vi "BMark_Create Tree.vi"(8 "error in (no error)":errorcluster, 9 "GroupByVI":bool, 10 "TreeRef":refnum<vi>, 11 "Bookmark info":T1[](array[typedef])) -> (0 "error out":errorcluster)   [LabVIEW 2017]
uses:
  controls/BMark_Bookmark Data.ctl
  controls/BMark_VI_Identifier.ctl
  <vilib>/addons/analyzer/_analyzerctrls.llb/VIAnCtl Analysis App Info.ctl
  globals/BMark_User Visible Strings.vi
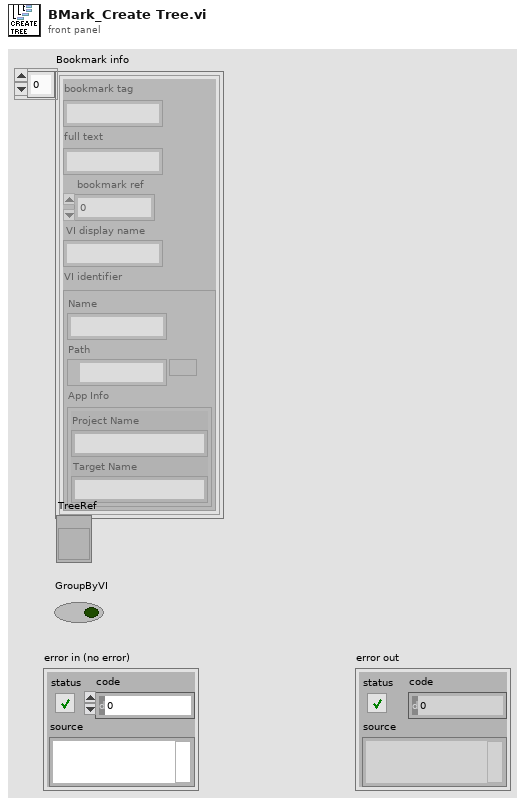
[diagram p1: front panel]
types:
  T1 = typedef "BMark_Bookmark Data.ctl" = cluster{"bookmark tag":string, "full text":string, "bookmark ref":i32, "VI display name":string, "VI identifier":T2}
  T2 = typedef "BMark_VI_Identifier.ctl" = cluster{"Name":string, "Path":path, "App Info":T3}
  T3 = typedef "VIAnCtl Analysis App Info.ctl" = cluster{"Project Name":string, "Target Name":string}
  T4 = enum8{"Enabled", "Disabled", "Disabled and Grayed Out"}
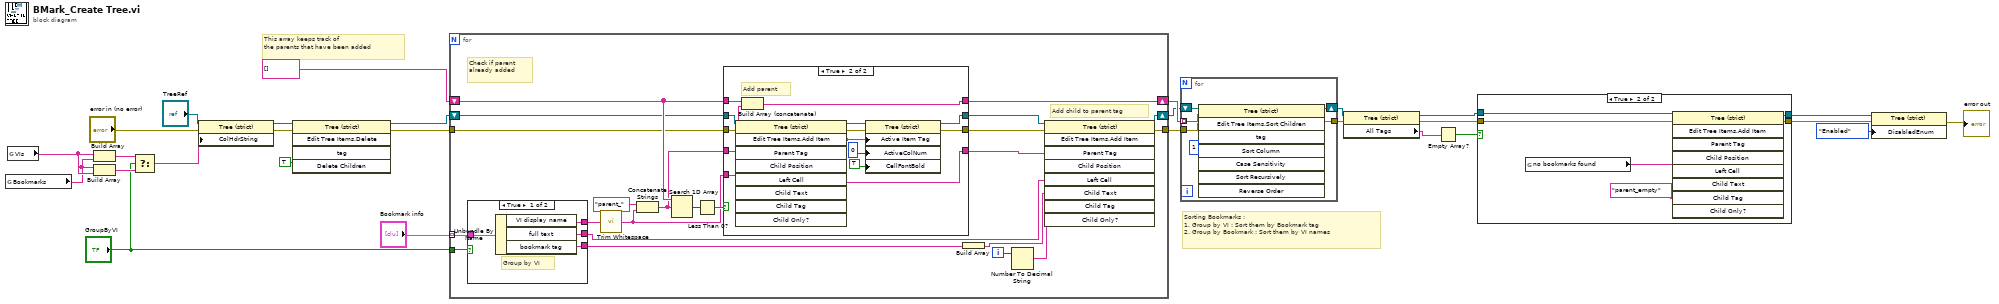
[diagram p0: block diagram]
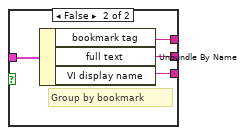
[diagram p2: hidden frame]
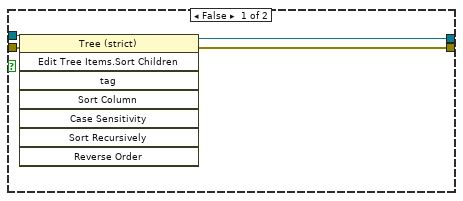
[diagram p4: hidden frame]
diagram:
  # "Sorting Bookmarks :\n1. Group by VI : Sort them by Bookmark tag\n2. Group by Bookmark : Sort them by VI names"
  # "This array keeps track of \nthe parents that have been added"
  n1 = global read "BMark_User Visible Strings.vi" "Bookmarks"() -> (w5:string)
  n2 = global read "BMark_User Visible Strings.vi" "VIs"() -> (w6:string)
  n3 = Build Array(w6, w5) -> (w18:string[])
  n4 = Build Array(w5, w6) -> (w17:string[])
  n5 = Select(t=w18, s="GroupByVI", f=w17) -> (s? t:f=w16:string[])
  n6 = property class="Tree (strict)"(reference="TreeRef", error in="error in (no error)", "ColHdrString"=w16) -> (reference out=w11:refnum<vi>, error out=w12:errorcluster)
  n7 = invoke class="Tree (strict)" method="Edit Tree Items.Delete"(reference=w11, error in=w12, "Delete Children"=TRUE ("Delete Children?")) -> (reference out=w26:refnum<vi>, error out=w27:errorcluster)  [unwired: 2 in, 3 out]
  n8 = for {
    tunnel: "Bookmark info" -> [w50] mode=indexing
    shift-right: [w46] -> w23
    shift-left: string[] [] -> [w47]
    tunnel: w27 -> [w33]
    tunnel: [w40] -> w22
    shift-right: [w38] -> w21
    shift-left: w26 -> [w45]
    tunnel: "GroupByVI" -> [w31]
    i -> [w35]
    # "Check if parent\nalready added"
    # "Add child to parent tag"
    n9 = case shown="True" w31 {
      tunnel: w50 -> [w54 w58]
      tunnel: [w53 w57] -> w41
      tunnel: [w52 w56] -> w30
      tunnel: [w51 w55] -> w32
      frame True {
        # "Group by VI"
        n10 = Unbundle By Name(w54) -> ("VI display name"=w52:string, "full text"=w53:string, "bookmark tag"=w51:string)
      }
      frame False {
        # "Group by bookmark"
        n11 = Unbundle By Name(w58) -> ("bookmark tag"=w56:string, "full text"=w57:string, "VI display name"=w55:string)
      }
    }
    n12 = call <vilib>:"Trim Whitespace.vi"("string"=w30) -> ("trimmed string"=w29:string)  [unwired: 1 in]
    n13 = Concatenate Strings("parent_", w29) -> (w37:string)
    n14 = Search 1D Array(1D array=w47, element=w37) -> (index of element=w49:i32)  [unwired: 1 in]
    n15 = Less Than 0?(x=w49) -> (x < 0?=w48:bool)
    n16 = case shown="True" w48 {
      tunnel: w47 -> [w62 w75]
      tunnel: w37 -> [w59 w68]
      tunnel: [w62 w74] -> w46
      tunnel: w33 -> [w60 w72]
      tunnel: [w60 w65] -> w36
      tunnel: w45 -> [w61 w73]
      tunnel: [w61 w64] -> w44
      tunnel: [w59 w63] -> w42
      tunnel: w29 -> [_ w71]
      frame False {
        # "Tag previously added"
      }
      frame True {
        # "Add parent"
        n17 = invoke class="Tree (strict)" method="Edit Tree Items.Add Item"(reference=w73, error in=w72, "Left Cell"=w71, "Child Tag"=w68) -> (reference out=w70:refnum<vi>, error out=w69:errorcluster, "Edit Tree Items:Add Item"=w63:string)  [unwired: 5 in, 6 out]
        n18 = Build Array (concatenate)(w75, w68) -> (w74:string[])
        n19 = property class="Tree (strict)"(reference=w70, error in=w69, "Active Item Tag"=w63, "ActiveColNum"=0 ("Active Cell:Active Column Number"), "CellFontBold"=TRUE ("Active Cell:Cell Font:Bold")) -> (reference out=w64:refnum<vi>, error out=w65:errorcluster)
      }
    }
    n20 = Build Array(w32) -> (w43:string[])
    n21 = Number To Decimal String(number=w35) -> (decimal integer string=w34:string)  [unwired: 1 in]
    n22 = invoke class="Tree (strict)" method="Edit Tree Items.Add Item"(reference=w44, error in=w36, "Parent Tag"=w42, "Left Cell"=w41, "Child Text"=w43, "Child Tag"=w34) -> (reference out=w38:refnum<vi>, error out=w40:errorcluster)  [unwired: 3 in, 7 out]
  }
  n23 = for {
    tunnel: w23 -> [w80] mode=indexing
    tunnel: [w79] -> w9
    tunnel: w22 -> [w77]
    shift-right: [w78] -> w10
    shift-left: w21 -> [w81]
    n24 = invoke class="Tree (strict)" method="Edit Tree Items.Sort Children"(reference=w81, error in=w77, "tag"=w80, "Sort Column"=1) -> (reference out=w78:refnum<vi>, error out=w79:errorcluster)  [unwired: 4 in, 6 out]
  }
  n25 = property class="Tree (strict)"(reference=w10, error in=w9) -> (reference out=w20:refnum<vi>, error out=w19:errorcluster, "All Tags"=w8:string[])
  n26 = Empty Array?(array=w8) -> (empty?=w7:bool)
  n27 = case shown="True" w7 {
    tunnel: w20 -> [w85 w91]
    tunnel: w19 -> [w84 w90]
    tunnel: [w83 w89] -> w3
    tunnel: [w82 w86] -> w4
    frame False {
      n28 = invoke class="Tree (strict)" method="Edit Tree Items.Sort Children"(reference=w85, error in=w84) -> (reference out=w82:refnum<vi>, error out=w83:errorcluster)  [unwired: 6 in, 6 out]
    }
    frame True {
      n29 = global read "BMark_User Visible Strings.vi" "no bookmarks found"() -> (w87:string)
      n30 = invoke class="Tree (strict)" method="Edit Tree Items.Add Item"(reference=w91, error in=w90, "Left Cell"=w87, "Child Tag"="parent_empty") -> (reference out=w86:refnum<vi>, error out=w89:errorcluster)  [unwired: 5 in, 7 out]
    }
  }
  n31 = property class="Tree (strict)"(reference=w4, error in=w3, "DisabledEnum"=T4."Enabled" ("Disabled")) -> (error out=→"error out":errorcluster)  [unwired: 1 out]
